vi "DeQueue.vi"   [LabVIEW 2013]
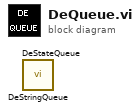
[diagram p0: block diagram]
diagram:
  n1 = call "DeStringQueue.vi"() -> ()  [unwired: 9 in, 3 out]
  n2 = call "DeStateQueue.vi"() -> ()  [unwired: 9 in, 3 out]
